vi "Configure Device.vi"(8 "error in":errorcluster, 11 "Vaisala Probe in":refnum<class "Vaisala.lvclass">) -> (0 "error out":errorcluster, 3 "Vaisala Probe out":refnum<class "Vaisala.lvclass">, 4 "SP":dbl, 5 "Settable?":bool)   [LabVIEW 2018, in "Vaisala Library.lvlib" / "Vaisala.lvclass"]
doc: "Configure the current instance of the Vaisala probe. In this case, we will get the correct address and then set the serial delayso that the probe responds in the correct amount of time. When configuration is done, make sure the session is closed."
uses:
  Vaisala.lvclass
  <vilib>/Utility/config.llb/NI_LVConfig.lvlib
  <vilib>/Utility/config.llb/Read Key (I32).vi
  reusable/Session APIs/Session Log/System Log.lvclass
  reusable/Session APIs/Serial/Serial Session.lvclass
  reusable/Session APIs/File Access/Config Data/Config Data.lvclass
  <vilib>/Utility/config.llb/Read Key (String).vi
  Configurable Device/Configurable Device.lvclass
  C:/Program Files (x86)/National Instruments/LabVIEW 2018/user.lib/_Session Fwk/Session - Root.lvclass
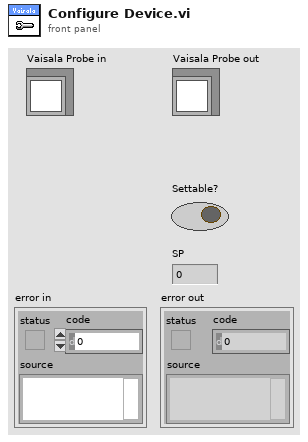
[diagram p1: front panel]
types:
  T1 = typedef "Config Data.lvclass/Config Session.ctl" = refnum<data-value>
  T2 = typedef "Session - Root.lvclass/Session Handle.ctl" = refnum<data-value>
  T3 = typedef "Serial Session.lvclass/Session Handle.ctl" = refnum<data-value>
  T4 = typedef "NI_LVConfig.lvlib/Config Data RefNum.ctl" = refnum<k1>
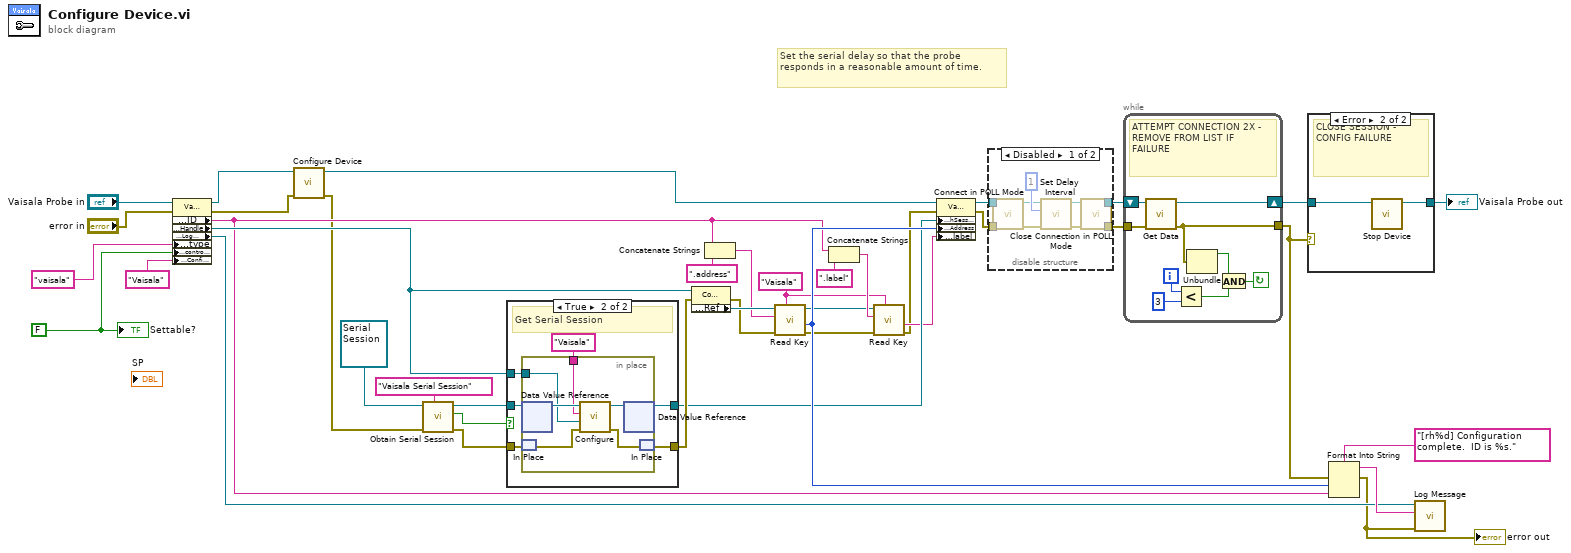
[diagram p0: block diagram]
diagram:
  w19 = FALSE ("controller_")
  w15 = "Vaisala" ("section")
  # "Set the serial delay so that the probe responds in a reasonable amount of time."
  n1 = property class="Vaisala"(reference="Vaisala Probe in", error in="error in", "Accessors:type"="vaisala" ("type"), "Accessors:controller_"=w19, "Accessors:Config Section"="Vaisala" ("section")) -> (reference out=w6:refnum<class "Vaisala.lvclass">, error out=w5:errorcluster, "Accessors:ID"=w10:string, "Accessors:Handle"=w29:T1, "Accessors:Log Session"=w30:T2)
  n2 = call-parent "Configure Device.vi"("error in"=w5, "Device in"=w6) -> ("error out"=w4:errorcluster, "Device out"=w3:refnum<class "Vaisala.lvclass">)  [unwired: 6 in, 2 out]
  n3 = call "Obtain Serial Session.vi"("Session Name ()"="Vaisala Serial Session", "error in"=w4, "Serial Session in"=refnum<class "Serial Session.lvclass"> refnum) -> ("error out"=w32:errorcluster, "created new?"=w33:bool, "hSerial"=w35:T3)  [unwired: 6 in]
  n4 = case shown="True" w33 {
    tunnel: w35 -> [w43 w49]
    tunnel: w32 -> [w42 w46]
    tunnel: [w43 w48] -> w27
    tunnel: [w42 w45] -> w31
    tunnel: w29 -> [_ w47]
    frame False {
    }
    frame True {
      # "Get Serial Session"
      n5 = in-place {
        in-place-border: w47 -> [w50]
        in-place-border: "Vaisala" ("section") -> [w51]
        n6 = in-place-dvr #1(w49) -> (w55:refnum<class "Serial Session.lvclass">)  [unwired: 1 out]
        n7 = in-place-match #2(w46) -> (w54:errorcluster)
        n8 = call "Configure.vi"("error in"=w54, "Config Handle"=w50, "section"=w51, "Serial Session in"=w55) -> ("error out"=w53:errorcluster, "Serial Session out"=w52:refnum<class "Serial Session.lvclass">)  [unwired: 6 in]
        n9 = in-place-dvr #1(w52) -> (w48:T3)  [unwired: 1 out]
        n10 = in-place-match #2(w53) -> (w45:errorcluster)
      }
    }
  }
  n11 = property class="Config Data"(reference=w29, error in=w31) -> (error out=w28:errorcluster, "Accessors:Ref"=w41:T4)  [unwired: 1 out]
  n12 = Concatenate Strings(w10, ".address" ("string")) -> (w16:string)
  n13 = call-poly <vilib>:"Read Key.vi"("section"=w15, "error in (no error)"=w28, "key"=w16, "refnum"=w41) -> ("error out"=w12:errorcluster, "value"=w34:i32, "refnum out"=w14:T4)  [unwired: 4 in, 1 out]
  n14 = Concatenate Strings(w10, ".label" ("string")) -> (w17:string)
  n15 = call-poly <vilib>:"Read Key.vi"("section"=w15, "error in (no error)"=w12, "key"=w17, "refnum"=w14) -> ("error out"=w11:errorcluster, "value"=w13:string)  [unwired: 4 in, 2 out]
  n16 = property class="Vaisala"(reference=w3, error in=w11, "Accessors:hSession"=w27, "Accessors:Address"=w34, "Accessors:label"=w13) -> (reference out=w25:refnum<class "Vaisala.lvclass">, error out=w26:errorcluster)
  n17 = disable-structure shown="Disabled" {
    disable-tunnel: w26 -> [w58 w64]
    disable-tunnel: w25 -> [w57 w65]
    disable-tunnel: [w56 w65] -> w24
    disable-tunnel: [_ w64] -> w9
    frame Disabled {
      n18 = call "Connect in POLL Mode.vi"("error in"=w58, "Vaisala in"=w57) -> ("error out"=w61:errorcluster, "Vaisala out"=w62:refnum<class "Vaisala.lvclass">)  [unwired: 8 in]
      n19 = call "Set Delay Interval.vi"("error in"=w61, "Delay In"=u8 1, "Vaisala in"=w62) -> ("error out"=w59:errorcluster, "Vaisala out"=w60:refnum<class "Vaisala.lvclass">)  [unwired: 7 in]
      n20 = call "Close Connection in POLL Mode.vi"("error in"=w59, "Vaisala in"=w60) -> ("Vaisala out"=w56:refnum<class "Vaisala.lvclass">)  [unwired: 8 in, 1 out]
    }
    frame Enabled {
    }
  }
  n21 = while {
    shift-right: [w72] -> w1
    shift-left: w24 -> [w71]
    tunnel: [w67] -> w23
    tunnel: w9 -> [w66]
    i -> [w74]
    stop <- w68 continue-if-true
    # "ATTEMPT CONNECTION 2X - REMOVE FROM LIST IF FAILURE"
    n22 = call-dynamic "Get Data.vi"("error in"=w66, "Cfg Dev in"=w71) -> ("error out"=w67:errorcluster, "Cfg Dev out"=w72:refnum<class "Vaisala.lvclass">)  [unwired: 7 in, 1 out]
    n23 = Less?(x=w74, y=3) -> (x < y?=w69:bool)
    n24 = Unbundle(w67) -> ("status"=w70:bool)  [unwired: 2 out]
    n25 = And(x=w70, y=w69) -> (x .and. y?=w68:bool)
  }
  n26 = case shown="Error" w23 {
    tunnel: w1 -> [w75 w77]
    tunnel: [w75 w76] -> w22
    frame No Error {
    }
    frame Error {
      # "CLOSE SESSION - CONFIG FAILURE"
      n27 = call-dynamic "Stop Device.vi"("Cfg Dev in"=w77) -> ("Cfg Dev out"=w76:refnum<class "Vaisala.lvclass">)  [unwired: 9 in, 1 out]
    }
  }
  "Vaisala Probe out" <- w22
  n28 = Format Into String(format string="[rh%d] Configuration complete.  ID is %s.", error in=w23, w34, w10) -> (resulting string=w38:string, error out=w21:errorcluster)  [unwired: 1 in]
  "error out" <- w21
  n29 = call "Log Message.vi"("error in"=w21, "MSG In"=w38, "session in"=w30) -> ()  [unwired: 7 in, 2 out]
  "Settable?" <- w19
